vi "Convert EOLs (String Array)__ogtk.vi"(9 "Convert to:":enum16{"CR", "LF", "CRLF"}(ring), 10 "String in":string[](array[string])) -> (1 "String out":string[](array[string]))   [LabVIEW 2020]
doc: "Converts all EOLs in the string to the type specified. A CRLF pair (\\r\\n) is considered to be one EOL. Therefore all CRLF pairs may be converted to just a CR or just a LF. Likewise single CRs or LFs may be converted to CRLF pairs. LabVIEW's Write File VIs have this option built into them, but Serial, TCP-IP, and others do not. There is no way to \"escape\" a CR, LF, or CRLF as not an EOL so be careful when using this utility."
panel:
  # "[OpenG VI Tags] ***Do Not Remove***"
  # "Convert EOLs.vi\n\nConverts all EOLs in the string to the type specified.\n\nPlease visit http://www.OpenG.org to learn about the\nOpen Source LabVIEW software movement.\n\nNOTICE -- YOU MUST LEAVE THIS NOTICE IN PLACE.  PER THE TERMS OF THE LICENSE BELOW, YOU MAY SUBLICENSE THIS SOFTWARE \nIN ANY WAY THAT DOES NOT CONFLICT WITH THIS LICENSE.\n\n### BSD License (http://www.opensource.org/licenses/bsd-license.php) Begin ###\n \nCopyright (c) 2002-2006, Jim Kring <jim@jimkring.com>\nCopyright (c) 2002, Cal-Bay Systems, Inc. <info@calbay.com>\n\nAll rights reserved.\n\nRedistribution and use in source and binary forms, with or without modification, are permitted provided that the following conditions are met:\n\n    * Redistributions of source code must retain the above copyright notice, this list of conditions and the following disclaimer.\n    * Redistributions in binary form must reproduce the above copyright notice, this list of conditions and the following disclaimer in the \n       documentation and/or other materials provided with the distribution.\n    * Neither the name of SciWare, James Kring, Inc., nor the names of its contributors may be used to endorse or promote products derived \n       from this software without specific prior written permission.\n\nTHIS SOFTWARE IS PROVIDED BY THE COPYRIGHT HOLDERS AND CONTRIBUTORS \"AS IS\" AND ANY EXPRESS OR IMPLIED WARRANTIES, \nINCLUDING, BUT NOT LIMITED TO, THE IMPLIED WARRANTIES OF MERCHANTABILITY AND FITNESS FOR A PARTICULAR PURPOSE ARE \nDISCLAIMED. IN NO EVENT SHALL THE COPYRIGHT OWNER OR CONTRIBUTORS BE LIABLE FOR ANY DIRECT, INDIRECT, INCIDENTAL,\n SPECIAL, EXEMPLARY, OR CONSEQUENTIAL DAMAGES (INCLUDING, BUT NOT LIMITED TO, PROCUREMENT OF SUBSTITUTE GOODS OR \nSERVICES; LOSS OF USE, DATA, OR PROFITS; OR BUSINESS INTERRUPTION) HOWEVER CAUSED AND ON ANY THEORY OF LIABILITY, \nWHETHER IN CONTRACT, STRICT LIABILITY, OR TORT (INCLUDING NEGLIGENCE OR OTHERWISE) ARISING IN ANY WAY OUT OF THE USE \nOF THIS SOFTWARE, EVEN IF ADVISED OF THE POSSIBILITY OF SUCH DAMAGE.\n\n### BSD License End ###"
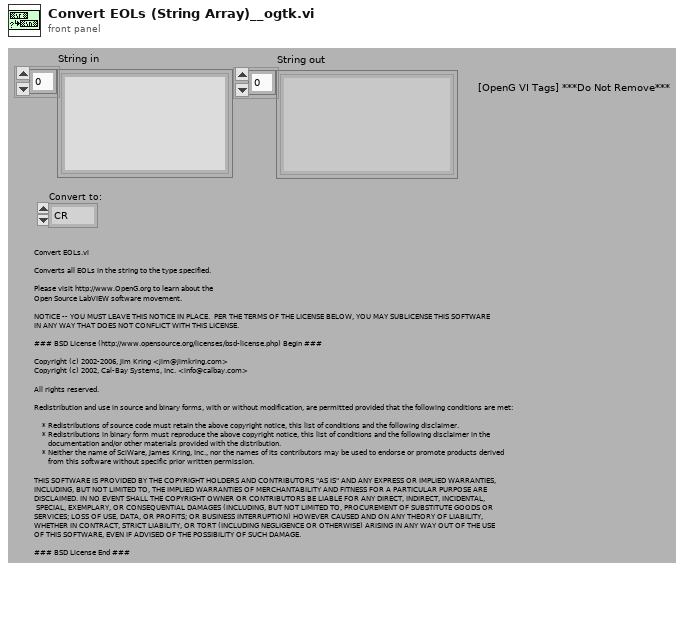
[diagram p1: front panel]
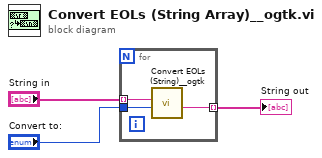
[diagram p0: block diagram]
diagram:
  n1 = for {
    tunnel: "Convert to:" -> [w6]
    tunnel: "String in" -> [w5] mode=indexing
    tunnel: [w4] -> w1 mode=indexing
    n2 = call <userlib>:"Convert EOLs (String)__ogtk.vi"("Convert to:"=w6, "String in"=w5) -> ("String out"=w4:string)  [unwired: 9 in]
  }
  "String out" <- w1
